vi "SR430.set bin width.vi"(0 "i ref in":refnum<vi>, 2 "binWidth [us]":dbl format="%.2f", 5 "error in (no error)":errorcluster) -> (14 "i ref out":refnum<vi>, 16 "actBinWidth [us]":dbl format="%.2f", 19 "error out":errorcluster)   [LabVIEW 2014, in "SR430.lvlib"]
doc: "Sets the bin width at the SR430. The allowed values are listed below. If the value is in between one of the listed values, the value is rounded to the next lower value. The bin width must be within 5ns < x < 10.486ms.\n\n5ns\n40ns\n80ns\n160ns\n320ns\n640ns\n1.28us\n2.56us\n5.12us\n10.24us\n20.48us\n40.96us\n81.92us\n163.84us\n327.68us\n655.36us\n1.3107ms\n2.6214ms\n5.2429ms\n10.486ms"
uses:
  SR430.lvlib
  CS_Core/CSApplicationBaseClasses/MCSBase/MCSBase.directionType.ctl
  CS_Core/CSApplicationBaseClasses/MCSBase/MCSBase.serviceType.ctl
  CSlibraries/UtilityLib/UtilityLib.valueStatus.ctl
  CS_Core/CSSystem/CoreDefs/CoreDefs.error_type.ctl
  instr.lib/SR430/SR430Driver.lvlib
  CS_Core/CSSystem/CoreLib/CoreLib.lvlib
  CS_Core/CSApplicationBaseClasses/MCSBase/MCSBase.lvlib
  CSlibraries/UtilityLib/UtilityLib.lvlib
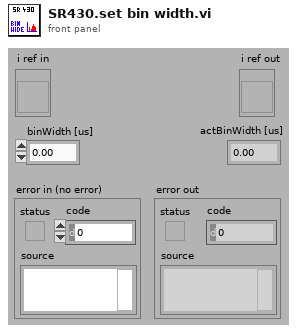
[diagram p1: front panel]
types:
  T1 = typedef "UtilityLib.lvlib/UtilityLib.valueStatus.ctl" = enum16{"no info available", "stand by/off", "on", "warning", "alarm/malfunction", "not implemented", "user action required", "important information", "system default", "control default", "indicator default", "button default"}
  T2 = typedef "MCSBase.lvlib/MCSBase.serviceType.ctl" = enum16{"counts", "totalCounts", "binWidth", "nOfBins", "nOfRecords", "status", "discrLevel", "discrSlope", "triggerLevel", "triggerSlope"}
  T3 = typedef "MCSBase.lvlib/MCSBase.directionType.ctl" = enum16{"unknown", "update actual value", "update nominal value", "update both"}
  T4 = typedef "CoreDefs.error_type.ctl" = enum16{"no error", "can't load process", "can't unload process", "process does not exist", "can't install process", "can't remove process", "unknown function", "time out", "can't execute function", "duplicate queue name", "super not found", "caller queue invalid", "can't ping process", "unknown error", "VISA Error", "VISA timeout", "GPIB timeout", "GPIB error", "communication error", "data type mismatch", "can't read data from OPC server", "can't write data to OPC server", "OET error", "function not implemented", "process already exists", "invalid Shared Variable name", "error writing Shared Variable", "error reading Shared Variable", "invalid client name", "corrupt database", "unknown class", "call not authorized", "parameter out of range", "OET timeout: can't get data to modify", "invalid queue name", "requested operation incompatible with current state", "event undefined", "event disabled", "state undefined", "caller is not a friend", "EventBuilder: bad eventID", "EventBuilder: no DAQ devices", "a thread must not stop itself", "UNUSED ELEMENT4", "DiscArchiver: eventData incomplete", "DiscArchiver: eventData does not belong to run", "DiscArchiver: can't open file", "DiscArchiver: can't write to file", "DiscArchiver: available disc space low", "can't acquire semaphore", "error reading data from database", "notifier object is not existing", "can't register process", "can't unregister process", "illegal event type", "object disabled", "object already exists", "can't change state", "Instrument not found", "no connection to remote node", "invalid reference", "N/A", "UNUSED ELEMENT 1", "element not found", "illegal TCP/IP connection detected", "object does not exist", "invalid access ID", "unknown CS system", "invalid privilige", "unsupported data type", "unsupported server type", "IO server already exists", "Shared Variable already exists"}
  T5 = typedef "SR430Driver.lvlib/SR430_VISA Control.ctl" = cluster{"VISA resource name":refnum<visa-resource-name>}
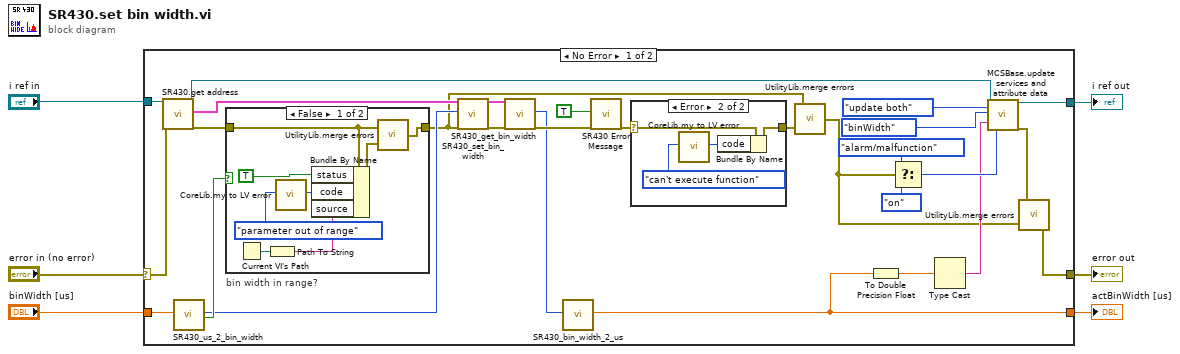
[diagram p0: block diagram]
diagram:
  n1 = case shown="No Error" "error in (no error)" {
    selector: "error in (no error)" -> [w20 w49]
    tunnel: "i ref in" -> [w34 w50]
    tunnel: "binWidth [us]" -> [w31 _]
    tunnel: [w7 w49] -> w4
    tunnel: [w12 w50] -> w3
    tunnel: [w9 _] -> w2
    frame No Error {
      n2 = call "SR430.get address.vi"("i ref in"=w34, "error in (no error)"=w20) -> ("i ref out"=w11:refnum<vi>, "address"=w33:T5, "error out"=w32:errorcluster)  [unwired: 15 in]
      n3 = call "SR430_us_2_bin_width.vi"("bin width [us]"=w31) -> ("binWidth"=w28:i32, "InRange?"=w29:bool)  [unwired: 16 in, 1 out]
      n4 = case "bin width in range?" shown="False" w29 {
        tunnel: w32 -> [w36 w43]
        tunnel: [w39 w43] -> w22
        frame False {
          n5 = Current VI's Path() -> (path=w38:path)
          n6 = Path To String(path=w38) -> (string=w37:string)
          n7 = call "CoreLib.my to LV error.vi"("ErrorTypes"=CoreDefs.error_type."parameter out of range") -> ("LV error code"=w41:i32)  [unwired: 17 in, 1 out]
          n8 = Bundle By Name(cluster=w36, "status"=TRUE, "code"=w41, "source"=w37) -> (w35:errorcluster)
          n9 = call "UtilityLib.merge errors.vi"("error2 (no error)"=w35, "error1 (no error)"=w36) -> ("error out"=w39:errorcluster)
        }
        frame True {
        }
      }
      n10 = call "SR430_set_bin_width.vi"("address"=w33, "binWidth"=w28, "error in (no error)"=w22) -> ("address out"=w25:T5, "error out"=w27:errorcluster)  [unwired: 15 in]
      n11 = call "SR430_get_bin_width.vi"("address"=w25, "error in (no error)"=w27) -> ("bin width"=w24:i32, "error out"=w26:errorcluster)  [unwired: 15 in, 1 out]
      n12 = call "SR430_bin_width_2_us.vi"("bin width"=w24) -> ("binWidth [us]"=w9:dbl)  [unwired: 16 in, 2 out]
      n13 = call "SR430 Error Message.vi"("addMessageToSource"=TRUE ("add message to source"), "error in (no error)"=w26) -> ("error out"=w30:errorcluster)  [unwired: 14 in, 3 out]
      n14 = case shown="Error" w30 {
        selector: w30 -> [w44 w48]
        tunnel: [w44 w45] -> w21
        frame No Error {
        }
        frame Error {
          n15 = call "CoreLib.my to LV error.vi"("ErrorTypes"=CoreDefs.error_type."can't execute function") -> ("LV error code"=w47:i32)  [unwired: 17 in, 1 out]
          n16 = Bundle By Name(cluster=w48, "code"=w47) -> (w45:errorcluster)
        }
      }
      n17 = call "UtilityLib.merge errors.vi"("error2 (no error)"=w21, "error1 (no error)"=w22) -> ("error out"=w10:errorcluster)
      n18 = To Double Precision Float(number=w9) -> (double precision float=w8:dbl)
      n19 = Select(t=UtilityLib.valueStatus."alarm/malfunction", s=w10, f=UtilityLib.valueStatus."on" ("quality")) -> (s? t:f=w18:T1)
      n20 = Type Cast(x=w8) -> (*(type *) &x=w15:string)  [unwired: 1 in]
      n21 = call "MCSBase.update services and attribute data.vi"("i ref in"=w11, "direction"=MCSBase.directionType."update both", "service"=MCSBase.serviceType."binWidth", "value"=w15, "quality"=w18) -> ("i ref out"=w12:refnum<vi>, "error out"=w19:errorcluster)  [unwired: 12 in, 1 out]
      n22 = call "UtilityLib.merge errors.vi"("error2 (no error)"=w10, "error1 (no error)"=w19) -> ("error out"=w7:errorcluster)
    }
    frame Error {
    }
  }
  "error out" <- w4
  "i ref out" <- w3
  "actBinWidth [us]" <- w2
